vi "Apply LMS Filter.vi"(0 "reference in":refnum<class "AdvSigProc.lvclass">, 5 "error in (no error)":errorcluster, 7 "Reference Signal":i32, 9 "Response Signal":i32) -> (13 "Iterations.Current":i32, 14 "reference out":refnum<class "AdvSigProc.lvclass">, 19 "error out":errorcluster)   [LabVIEW 2022 SP3, in "AdvSigProc.lvclass"]
uses:
  AdvSigProc.lvclass
  API/GSwFormDSP_class/functions/Attribute Options.ctl
  <vilib>/addons/Adaptive Filters/Processing/AFT Filter Signal and Update Coefficients (Real, Waveform).vi
  <vilib>/addons/Adaptive Filters/Analysis/AFT Get Coefficients (FIR, Real).vi
  API/GSwFormDSP_class/GSwFormDSP.lvclass
  <vilib>/addons/Adaptive Filters/NI_AdaptiveFilter.lvlib
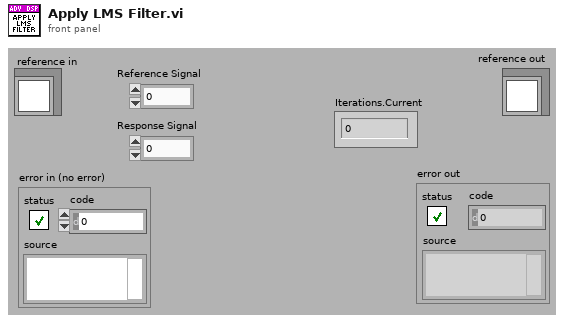
[diagram p1: front panel]
types:
  T1 = typedef "AdvSigProc.lvclass/ObjectAttributesRef.ctl" = refnum<data-value>
  T2 = typedef "AdvSigProc.lvclass/ObjectAttributes.ctl" = cluster{"Time Data":cluster{"New Time Data Obj?":bool, "GSwFormDSP":refnum<class "GSwFormDSP.lvclass">}, "LMS Parameters":T3}
  T3 = typedef "AdvSigProc.lvclass/LMS.ctl" = cluster{"adaptive filter Ref":refnum<k20>, "Filtered Signals":refnum<class "GSwFormDSP.lvclass">, "Filter Coefs":dbl[], "Input Parameters":T4, "Iteration Metrics":T5[]}
  T4 = typedef "AdvSigProc.lvclass/LMS Input Parameters.ctl" = cluster{"Type":enum16{"Normalized LMS", "LMS", "FIR Sign LMS", "FIR Fast Block LMS", "RLS", "QR - RLS"}, "Filter Class":enum16{"Noise Cancelling (BGN Ref)", "Noise Cancelling (Speech Ref)"}, "Filter Length":i32, "µ Parameters":cluster{"Type":enum16{"User Input", "Auto µ"}, "step size":dbl}, "Iterations":cluster{"Current":i32, "Maximum":i32}}
  T5 = typedef "AdvSigProc.lvclass/Iteration Metrics.ctl" = cluster{"Name":string, "Max":dbl, "Min":dbl, "Values History":dbl[]}
  T6 = typedef "GSwFormDSP.lvclass/Attribute Options.ctl" = enum16{"Append to Attribute using \"( )\"", "Replace Attribute Value"}
  T7 = enum16{"Noise Cancelling (BGN Ref)", "Noise Cancelling (Speech Ref)"}
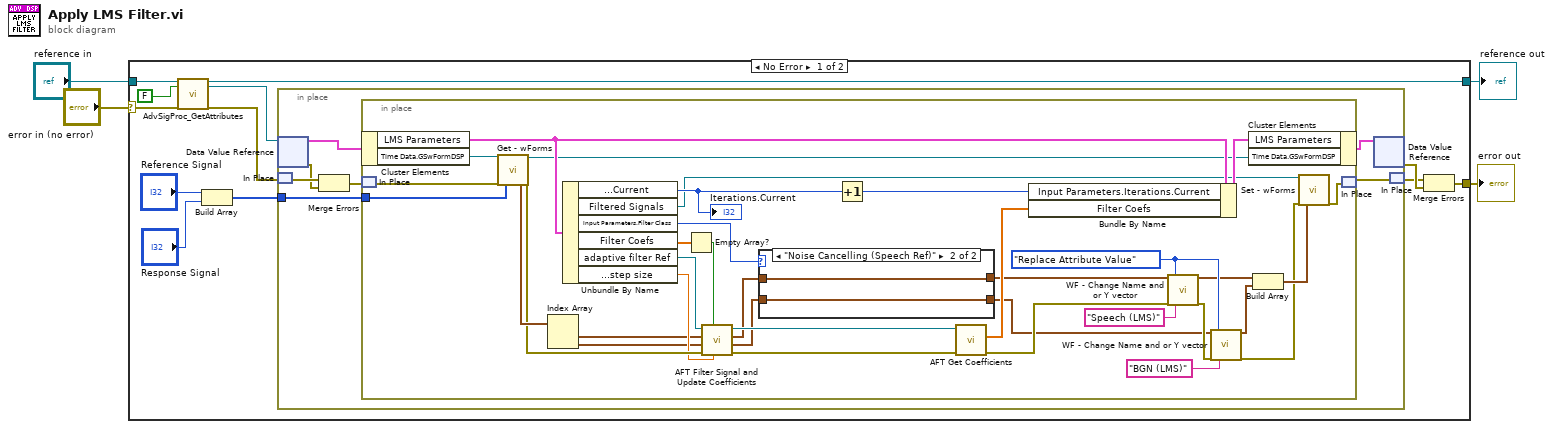
[diagram p0: block diagram]
diagram:
  n1 = case shown="No Error" "error in (no error)" {
    selector: "error in (no error)" -> [w12 w64]
    tunnel: [w16 w64] -> w3
    tunnel: [w11 w63] -> w1
    tunnel: "reference in" -> [w14 w63]
    frame No Error {
      n2 = call "AdvSigProc_GetAttributes.vi"("reference in"=w14, "return data? (T)"=FALSE, "error in (no error)"=w12) -> ("reference out"=w11:refnum<class "AdvSigProc.lvclass">, "attributes ref"=w10:T1, "error out"=w9:errorcluster)  [unwired: 13 in, 1 out]
      n3 = Build Array("Reference Signal", "Response Signal") -> (w5:i32[])
      n4 = in-place {
        in-place-border: w5 -> [w17]
        n5 = in-place-dvr #1(w10) -> (w22:T2, w20:errorcluster)
        n6 = in-place-match #2(w9) -> (w21:errorcluster)
        n7 = Merge Errors(w21, w20) -> (w19:errorcluster)
        n8 = in-place {
          in-place-border: w17 -> [w50]
          w40 = Attribute_Options."Replace Attribute Value" ("Attribute Option")
          n9 = in-place-cluster #3(w22) -> ("LMS Parameters"=w57:T3, "Time Data.GSwFormDSP"=w53:refnum<class "GSwFormDSP.lvclass">)
          n10 = in-place-match #4(w19) -> (w51:errorcluster)
          n11 = call-dynamic "Get - wForms.vi"("reference in"=w53, "error in (no error)"=w51, "Indexes (Empty = ALL)"=w50) -> ("wForms"=w49:waveform(dbl)[], "reference out"=w52:refnum<class "GSwFormDSP.lvclass">, "error out"=w39:errorcluster)  [unwired: 13 in, 1 out]
          n12 = Index Array(array=w49) -> (element #1=w32:waveform(dbl), element #2=w31:waveform(dbl))  [unwired: 2 in]
          n13 = Unbundle By Name(w57) -> ("Input Parameters.Iterations.Current"=w56:i32, "Filtered Signals"=w44:refnum<class "GSwFormDSP.lvclass">, "Input Parameters.Filter Class"=w48:T7, "Filter Coefs"=w54:dbl[], "adaptive filter Ref"=w38:refnum<k20>, "Input Parameters.µ Parameters.step size"=w37:dbl)
          "Iterations.Current" <- w56
          n14 = Empty Array?(array=w54) -> (empty?=w30:bool)
          n15 = call-poly <vilib>:"AFT Filter Signal and Update Coefficients.vi"("step size"=w37, "reset? (F)"=w30, "error in (no error)"=w39, "d(n)"=w31, "x(n)"=w32, "adaptive filter in"=w38) -> ("error out"=w35:errorcluster, "e(n)"=w28:waveform(dbl), "y(n)"=w29:waveform(dbl), "adaptive filter out"=w36:refnum<k20>)  [unwired: 2 in]
          n16 = case shown="\"Noise Cancelling (Speech Ref)\"" w48 {
            tunnel: [w60 w62] -> w24
            tunnel: w28 -> [w59 w62]
            tunnel: [w59 w61] -> w27
            tunnel: w29 -> [w60 w61]
            frame "Noise Cancelling (BGN Ref)", Default {
            }
            frame "Noise Cancelling (Speech Ref)" {
            }
          }
          n17 = Increment(x=w56) -> (x+1=w55:i32)
          n18 = call-poly <vilib>:"AFT Get Coefficients.vi"("error in (no error)"=w35, "adaptive filter in"=w36) -> ("error out"=w34:errorcluster, "coefficients"=w47:dbl[])  [unwired: 7 in, 1 out]
          n19 = Bundle By Name(cluster=w57, "Input Parameters.Iterations.Current"=w55, "Filter Coefs"=w47) -> (w58:T3)
          n20 = call "WF - Change Name and or Y vector.vi"("wForm IN"=w27, "error in (no error)"=w34, "Attribute Option"=w40, "SigName Update"="Speech (LMS)") -> ("wForm OUT"=w26:waveform(dbl), "error out"=w33:errorcluster)  [unwired: 14 in]
          n21 = call "WF - Change Name and or Y vector.vi"("wForm IN"=w24, "error in (no error)"=w33, "Attribute Option"=w40, "SigName Update"="BGN (LMS)") -> ("wForm OUT"=w25:waveform(dbl), "error out"=w42:errorcluster)  [unwired: 14 in]
          n22 = in-place-cluster #3("LMS Parameters"=w58, "Time Data.GSwFormDSP"=w52) -> (w23:T2)
          n23 = Build Array(w26, w25) -> (w43:waveform(dbl)[])
          n24 = call "Set - wForms.vi"("reference in"=w44, "error in (no error)"=w42, "wForms"=w43) -> ("error out"=w41:errorcluster)  [unwired: 15 in, 1 out]
          n25 = in-place-match #4(w41) -> (w18:errorcluster)
        }
        n26 = in-place-dvr #1(w23) -> (w15:errorcluster)  [unwired: 1 out]
        n27 = in-place-match #2(w18) -> (w8:errorcluster)
      }
      n28 = Merge Errors(w8, w15) -> (w16:errorcluster)
    }
    frame Error {
    }
  }
  "error out" <- w3
  "reference out" <- w1
